vi "Set busy.vi"(8 "error in (no error)":errorcluster, 10 "busy?":bool, 11 "Retiga in":refnum<class "Retiga.lvclass">) -> (0 "error out":errorcluster, 3 "Retiga out":refnum<class "Retiga.lvclass">)   [LabVIEW 2012, in "Retiga.lvclass"]
uses:
  Retiga.lvclass
  Retiga.lvclass/Retiga.ctl
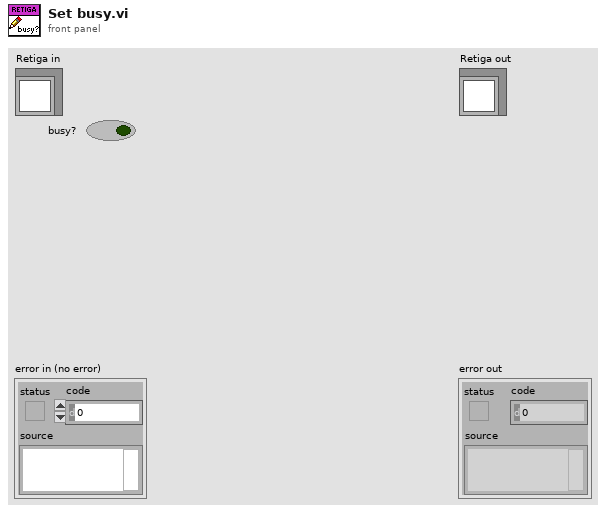
[diagram p1: front panel]
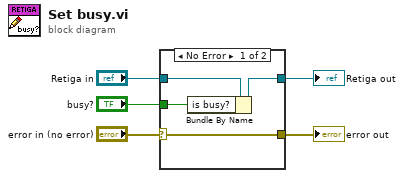
[diagram p0: block diagram]
diagram:
  n1 = case shown="No Error" "error in (no error)" {
    selector: "error in (no error)" -> [w9 w11]
    tunnel: [w9 w11] -> w4
    tunnel: [w7 w10] -> w2
    tunnel: "Retiga in" -> [w8 w10]
    tunnel: "busy?" -> [w6 _]
    frame No Error {
      n2 = Bundle By Name(cluster=w8, "is busy?"=w6) -> (w7:refnum<class "Retiga.lvclass">)
    }
    frame Error {
    }
  }
  "error out" <- w4
  "Retiga out" <- w2
